vi "Visa_in_out.vi"(8 "error in (no error)":errorcluster, 9 "read count":u32=256, 10 "write buffer":string, 11 "VISA resource name":refnum<visa-resource-name>) -> (0 "error out":errorcluster, 2 "read buffer":string, 3 "VISA resource name out":refnum<visa-resource-name>)   [LabVIEW 2015]
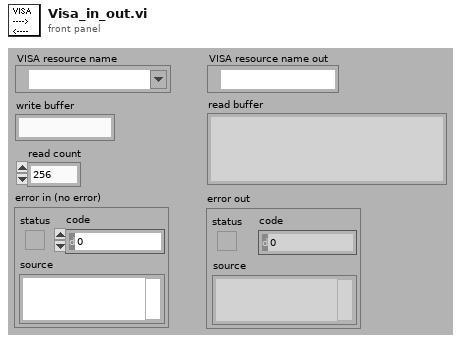
[diagram p1: front panel]
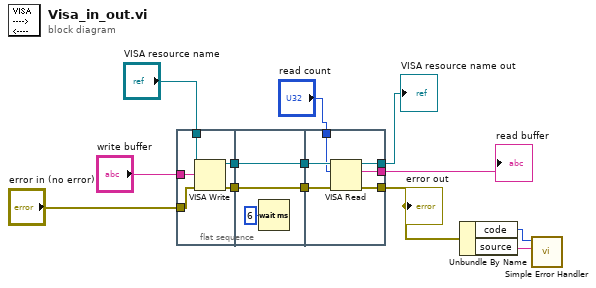
[diagram p0: block diagram]
diagram:
  n1 = flat-sequence {
    tunnel: "VISA resource name" -> [w18]
    tunnel: "error in (no error)" -> [w17]
    tunnel: "write buffer" -> [w14]
    tunnel: [w16] -> w10
    tunnel: [w15] -> w9
    tunnel: w10 -> [w21]
    tunnel: w9 -> [w20]
    tunnel: [w21] -> w8
    tunnel: [w20] -> w7
    tunnel: w8 -> [w26]
    tunnel: w7 -> [w27]
    tunnel: [w25] -> w3
    tunnel: [w24] -> w6
    tunnel: [w23] -> w5
    tunnel: "read count" -> [w22]
    frame #0 {
      n2 = VISA Write(VISA resource name=w18, write buffer=w14, error in (no error)=w17) -> (VISA resource name out=w15:refnum<visa-resource-name>, error out=w16:errorcluster)  [unwired: 1 out]
    }
    frame #1 {
      n3 = Wait (ms)(milliseconds to wait=u32 6) -> ()  [unwired: 1 out]
    }
    frame #2 {
      n4 = VISA Read(VISA resource name=w27, byte count=w22, error in (no error)=w26) -> (VISA resource name out=w23:refnum<visa-resource-name>, read buffer=w24:string, error out=w25:errorcluster)  [unwired: 1 out]
    }
  }
  n5 = Unbundle By Name(w3) -> ("code"=w2:i32, "source"=w1:string)
  n6 = call <vilib>:"Simple Error Handler.vi"("error code (no error:0)"=w2, "error source (\" \")"=w1) -> ()  [unwired: 2 in, 6 out]
  "error out" <- w3
  "VISA resource name out" <- w5
  "read buffer" <- w6
